vi "report generation  window.vi"(0 "connection reference":T1, 7 "error in":errorcluster) -> (4 "connection reference out":T1, 15 "error out":errorcluster)   [LabVIEW 2024]
uses:
  <vilib>/addons/database/Connection.llb/Conn ObjectReference.ctl
  <vilib>/Utility/miscctls.llb/LVRowAndColumnTypeDef.ctl
  Global variable.vi
  <vilib>/addons/database/Connection.llb/DB Tools Open Connec (String).vi
  Variable/Global.vi
  <vilib>/addons/database/NI_Database_API.lvlib
panel:
  in  "Final Barcode":string
  in  "Search by Laser 2":bool
  in  "Export":bool
  in  "Type of file":enum32{"Text", "Csv"}(radio)
  in  "Report File Name":string
  out "date/time string":string
  out "Result":string[][](table)
  in  "Exit":bool
  in  "Barcode":string
  in  "Search by Date":bool
  in  "model name selection":bool
  in  "MODEL":enum16{"NO Station", "Station 1", "Station 2"}(ring)
  in  "Search by Date":bool
  in  "To Date":timestamp format="%<%y/%m/%d>T"
  in  "From date":timestamp format="%<%y/%m/%d>T"
  out "exit":bool
  out "Numeric":i32
  # "TESTING DATALOGGING SYSTEM"
  # "REPORT SCREEN"
  # "to"
  # "Report  Genrate"
  # "A1234567B567001"
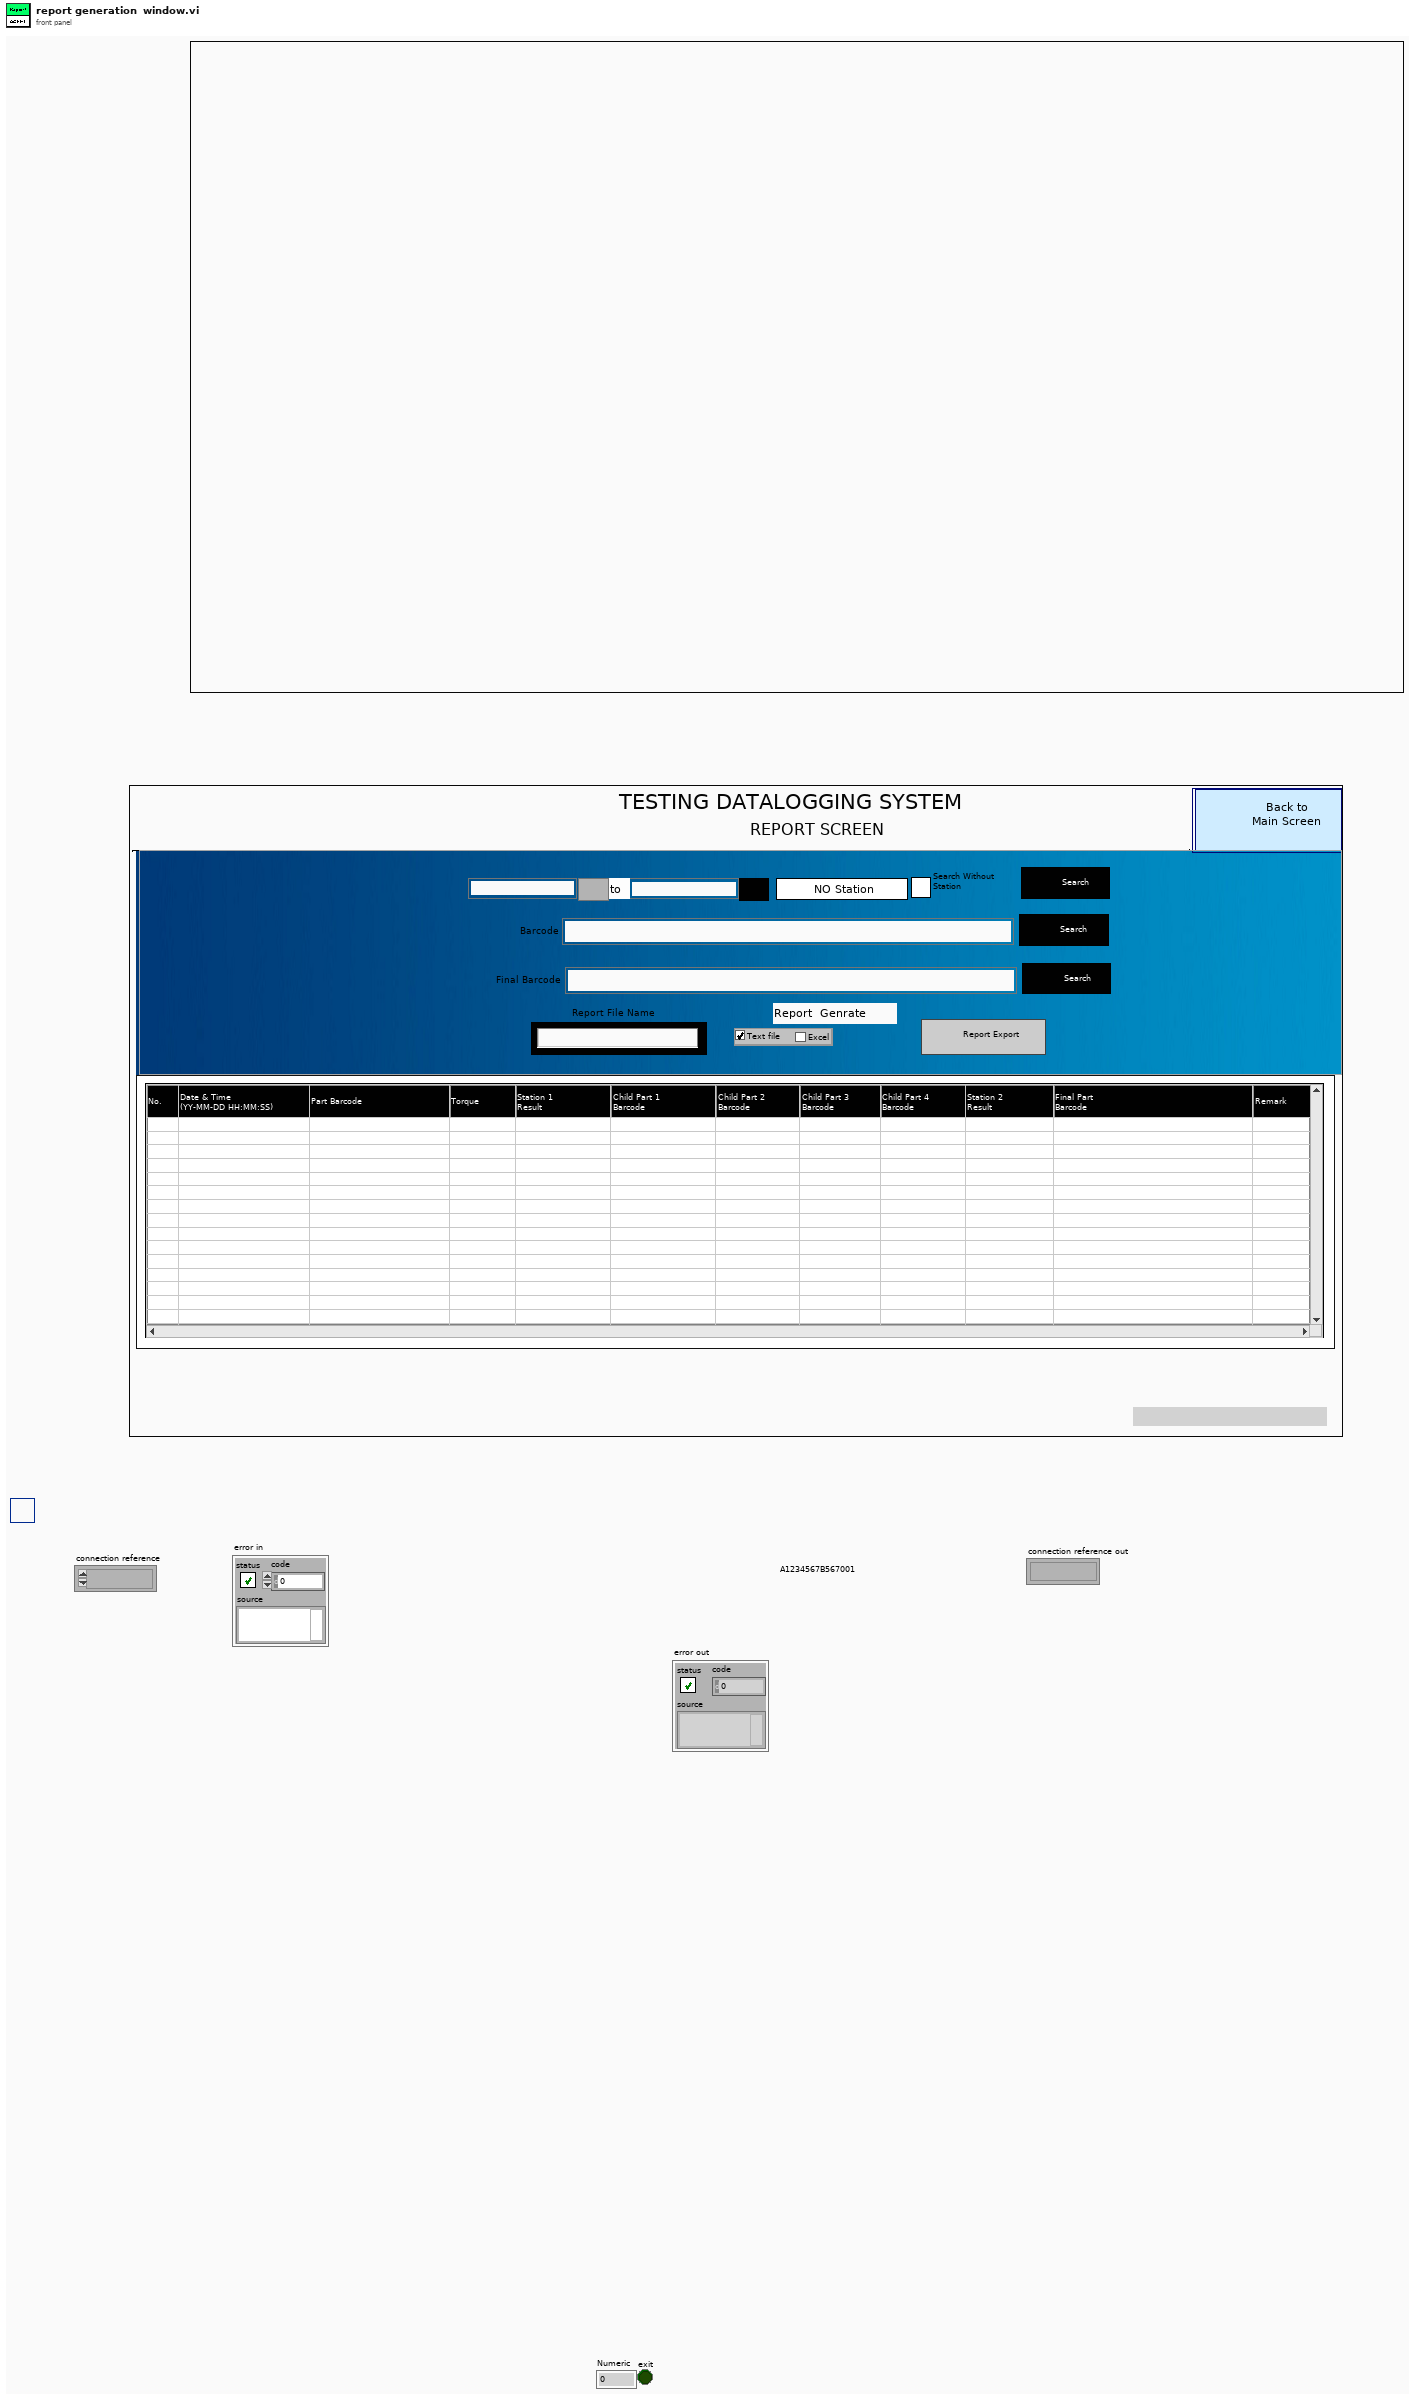
[diagram p1: front panel]
types:
  T1 = typedef "NI_Database_API.lvlib/Conn ObjectReference.ctl" = refnum<k1>
  T2 = typedef "LVRowAndColumnTypeDef.ctl" = cluster{"Row":i32, "Column":i32}
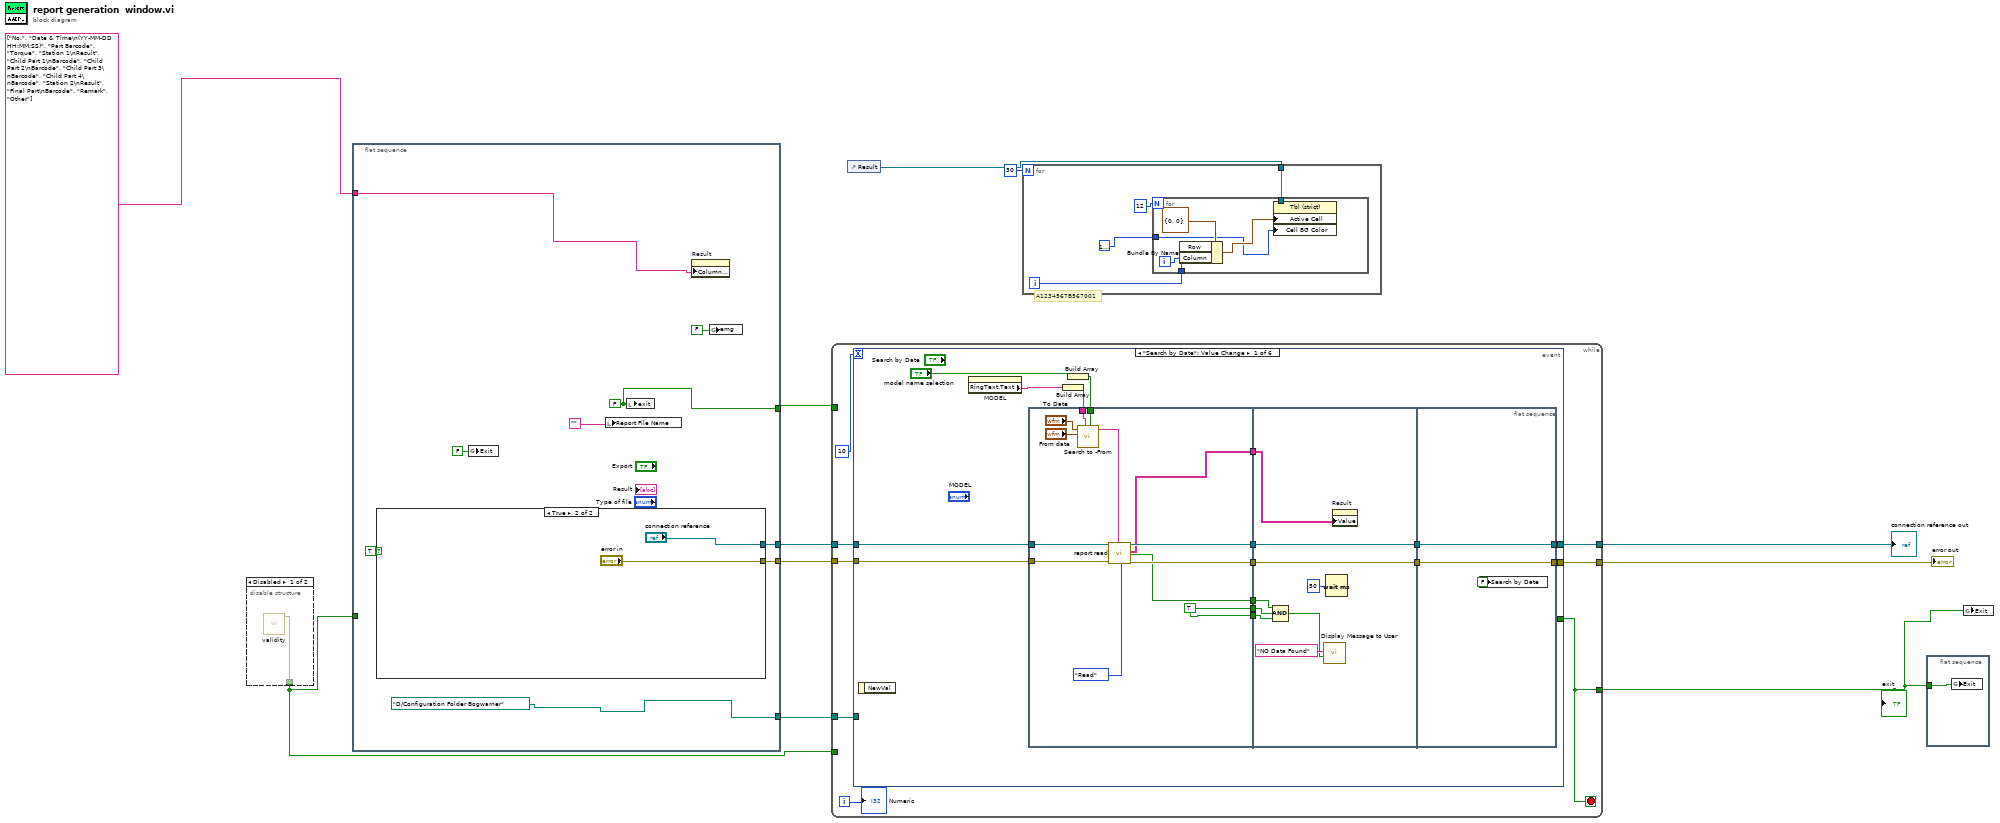
[diagram p0: block diagram]
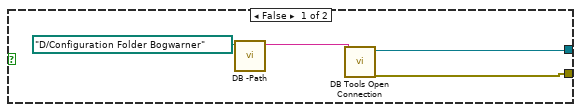
[diagram p3: hidden frame]
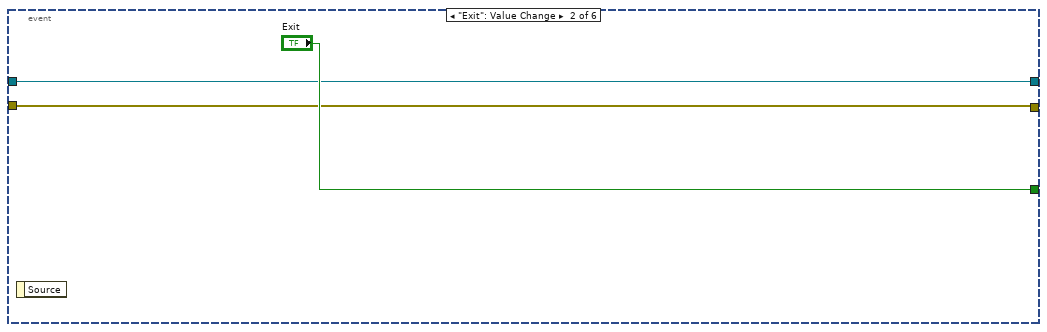
[diagram p4: hidden frame]
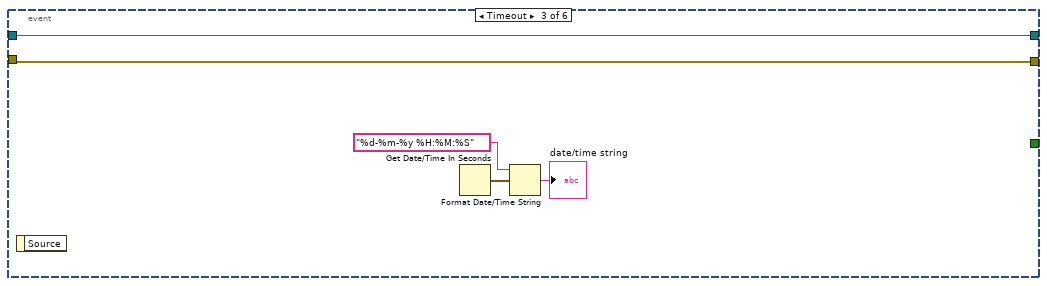
[diagram p5: hidden frame]
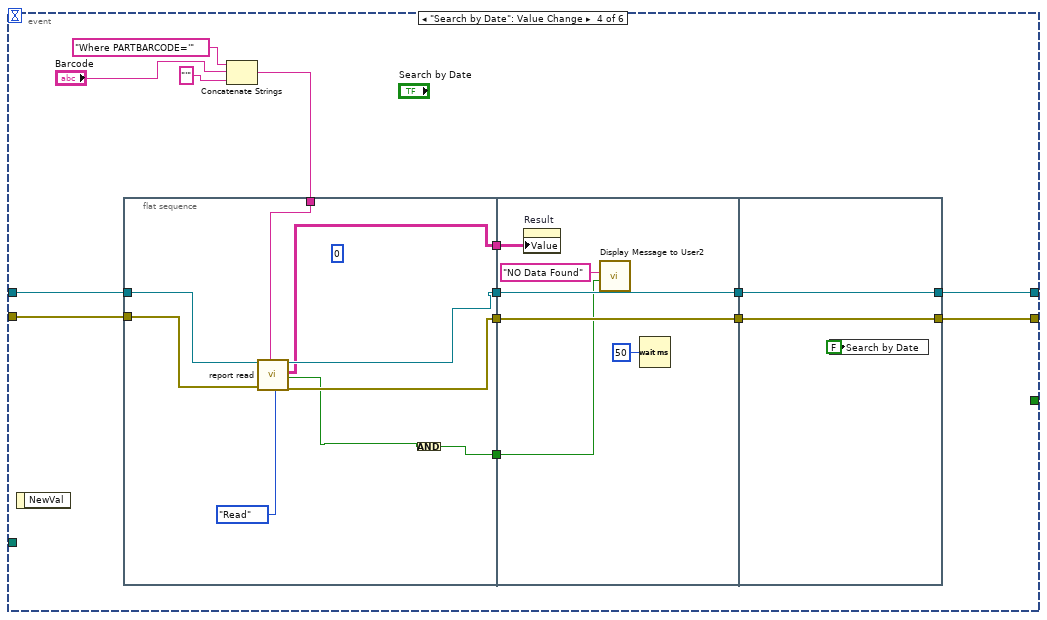
[diagram p6: hidden frame]
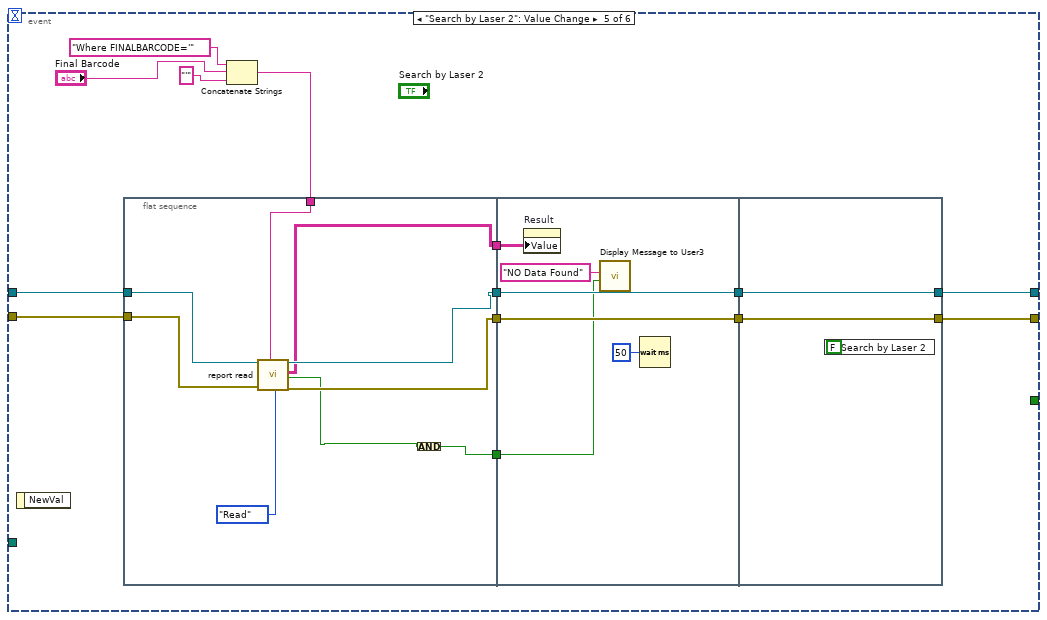
[diagram p7: hidden frame]
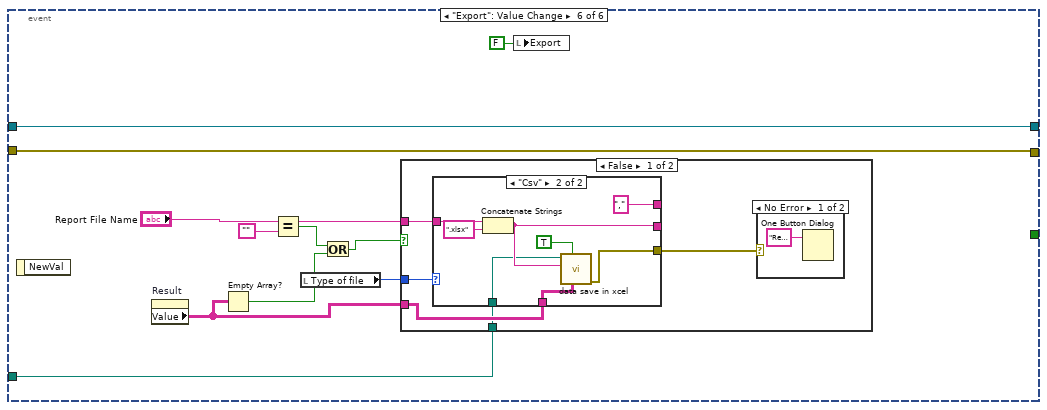
[diagram p8: hidden frame]
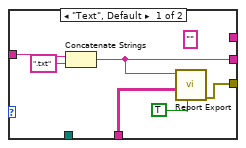
[diagram p10: hidden frame]
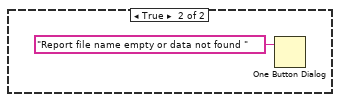
[diagram p11: hidden frame]
diagram:
  # "A1234567B567001"
  n1 = disable-structure shown="Disabled" {
    disable-tunnel: [w12 _] -> w6
    frame Disabled {
      n2 = call "validity.vi"() -> ("NOt valid"=w12:bool)  [unwired: 11 in]
    }
    frame Enabled {
    }
  }
  n3 = flat-sequence {
    tunnel: [w20] -> w10
    tunnel: [w18] -> w8
    tunnel: [w19] -> w7
    tunnel: w6 -> [_]
    tunnel: [path "D:/Configuration Folder Bogwarner" ("path")] -> w4
    tunnel: string[] ["No.", "Date & Time\n(YY-MM-DD HH:MM:SS)", "Part Barcode", "Torque", "Station 1\nResult", "Child Part 1\nBarcode", "Child Part 2\nBarcode", "Child Part 3\nBarcode", "Child Part 4\nBarcode", "Station 2\nResult", "Final Part\nBarcode", "Remark", "Other"] ("Column Header Strings[]") -> [w13]
    frame #0 {
      w20 = FALSE ("exit")
      n4 = case shown="True" TRUE {
        tunnel: [w23 "error in"] -> w19
        tunnel: [w22 "connection reference"] -> w18
        frame False {
          n5 = call "DB -Path.vi"("path"=path "D:/Configuration Folder Bogwarner") -> ("String"=w24:string)  [unwired: 8 in, 2 out]
          n6 = call-poly <vilib>:"DB Tools Open Connection.vi"("connection information"=w24) -> ("error out"=w23:errorcluster, "connection reference"=w22:T1)  [unwired: 7 in]
        }
        frame True {
        }
      }
      n7 = global write "Global variable.vi" "Exit"(FALSE ("Exit")) -> ()
      n8 = local write "Report File Name"("") -> ()
      n9 = local write "exit"(w20) -> ()
      n10 = property on="Result" class="Tbl (strict)"("Column Headers[]"=w13) -> ()  [unwired: 2 in, 2 out]
      n11 = global write "Global.vi" "emg"(FALSE ("emg")) -> ()
    }
  }
  n12 = while {
    tunnel: w8 -> [w35]
    tunnel: w7 -> [w34]
    tunnel: [w33] -> w11
    tunnel: [w32] -> w5
    tunnel: [w31] -> w9
    tunnel: w10 -> [_]
    tunnel: w6 -> [_]
    tunnel: w4 -> [w28]
    i -> [w30]
    stop <- w31 stop-if-true
    n13 = event shown="[0] \"Search by Date\": Value Change" {
      selector: _ -> [_ _ _ _ _ _]
      dyn-events: _ -> [_ _ _ _ _ _]
      timeout: 10 -> [_ _ _ _ _ _]
      tunnel: [_ "Exit" _ _ _ _] -> w31
      tunnel: w35 -> [w51 w78 w84 w98 w130 w159]
      tunnel: w34 -> [w50 w77 w83 w97 w129 w158]
      tunnel: [w49 w78 w84 w96 w128 w159] -> w33
      tunnel: [w48 w77 w83 w95 w127 w158] -> w32
      tunnel: w28 -> [_ _ _ _ _ w149]
      event "Search by Date": Value Change {
        n14 = event-data() -> ()  [unwired: 1 in, 1 out]
        n15 = property on="MODEL" class="Enum (strict)"() -> ("RingText.Text"=w40:string)  [unwired: 2 in, 2 out]
        n16 = flat-sequence {
          tunnel: w51 -> [w64]
          tunnel: w50 -> [w63]
          tunnel: [w60] -> w47
          tunnel: [w59] -> w46
          tunnel: w42 -> [w57]
          tunnel: w41 -> [w56]
          tunnel: [w54] -> w39
          tunnel: [w53] -> w38
          tunnel: [w53] -> w37
          tunnel: [w52] -> w36
          tunnel: w47 -> [w73]
          tunnel: w46 -> [w72]
          tunnel: [w73] -> w45
          tunnel: [w72] -> w44
          tunnel: w39 -> [w68]
          tunnel: w38 -> [w67]
          tunnel: w37 -> [w66]
          tunnel: w36 -> [w69]
          tunnel: [w75] -> w48
          tunnel: [w76] -> w49
          tunnel: w45 -> [w76]
          tunnel: w44 -> [w75]
          frame #0 {
            w53 = TRUE ("DMC TESTED:T")
            n17 = call "Search to -From.vi"("Enable"=w56, "Selection"=w57, "From date"="From date", "To Date"="To Date") -> ("search dataString"=w58:string)  [unwired: 6 in, 1 out]
            n18 = call "report read.vi"("connection reference"=w64, "error in (no error)"=w63, "search dataString"=w58, "Enum"=enum16{"Write", "Read"}."Read") -> ("connection reference out"=w60:T1, "Search result"=w52:string[][], "DMC TESTED:T"=w54:bool, "error out"=w59:errorcluster)  [unwired: 10 in, 2 out]
          }
          frame #1 {
            n19 = Compound Arithmetic op=AND(w68, w67, w66) -> (w65:bool)
            n20 = call "Display Message to User"("Enable"=w65, "Message"="NO Data Found") -> ()  [unwired: 8 in, 2 out]
            n21 = Wait (ms)(milliseconds to wait=u32 50) -> ()  [unwired: 1 out]
            n22 = property on="Result" class="Tbl (strict)"("Value"=w69) -> ()  [unwired: 2 in, 2 out]
          }
          frame #2 {
            n23 = local write "Search by Date"(FALSE ("Search")) -> ()
          }
        }
        n24 = Build Array(w40) -> (w42:string[])
        n25 = Build Array("model name selection") -> (w41:bool[])
      }
      event "Exit": Value Change {
        n26 = event-data() -> ()  [unwired: 1 in, 1 out]
      }
      event Timeout {
        n27 = event-data() -> ()  [unwired: 1 in, 1 out]
        n28 = Get Date/Time In Seconds() -> (seconds since 1Jan1904=w81:timestamp)
        n29 = Format Date/Time String(time format string (%c)="%d-%m-%y %H:%M:%S", seconds (now)=w81) -> (date/time string=→"date/time string":string)  [unwired: 1 in]
      }
      event "Search by Date": Value Change {
        n30 = event-data() -> ()  [unwired: 1 in, 1 out]
        n31 = flat-sequence {
          tunnel: w98 -> [w107]
          tunnel: w97 -> [w106]
          tunnel: [w103] -> w94
          tunnel: [w102] -> w93
          tunnel: w87 -> [w104]
          tunnel: [w100] -> w86
          tunnel: [w99] -> w85
          tunnel: w94 -> [w113]
          tunnel: w93 -> [w112]
          tunnel: [w113] -> w92
          tunnel: [w112] -> w91
          tunnel: w86 -> [w110]
          tunnel: w85 -> [w108]
          tunnel: [w115] -> w95
          tunnel: [w116] -> w96
          tunnel: w92 -> [w116]
          tunnel: w91 -> [w115]
          frame #0 {
            (unwired) 0 ("disabled index (col)")
            n32 = call "report read.vi"("connection reference"=w107, "error in (no error)"=w106, "search dataString"=w104, "Enum"=enum16{"Write", "Read"}."Read") -> ("connection reference out"=w103:T1, "Search result"=w99:string[][], "DMC TESTED:T"=w101:bool, "error out"=w102:errorcluster)  [unwired: 10 in, 2 out]
            n33 = Compound Arithmetic op=AND(w101) -> (w100:bool)
          }
          frame #1 {
            n34 = property on="Result" class="Tbl (strict)"("Value"=w108) -> ()  [unwired: 2 in, 2 out]
            n35 = call "Display Message to User2"("Enable"=w110, "Message"="NO Data Found") -> ()  [unwired: 8 in, 2 out]
            n36 = Wait (ms)(milliseconds to wait=u32 50) -> ()  [unwired: 1 out]
          }
          frame #2 {
            n37 = local write "Search by Date"(FALSE ("Search")) -> ()
          }
        }
        n38 = Concatenate Strings("Where PARTBARCODE='" ("string"), "Barcode", "'" ("string")) -> (w87:string)
      }
      event "Search by Laser 2": Value Change {
        n39 = event-data() -> ()  [unwired: 1 in, 1 out]
        n40 = flat-sequence {
          tunnel: w130 -> [w139]
          tunnel: w129 -> [w138]
          tunnel: [w135] -> w126
          tunnel: [w134] -> w125
          tunnel: w119 -> [w136]
          tunnel: [w132] -> w118
          tunnel: [w131] -> w117
          tunnel: w126 -> [w145]
          tunnel: w125 -> [w144]
          tunnel: [w145] -> w124
          tunnel: [w144] -> w123
          tunnel: w118 -> [w142]
          tunnel: w117 -> [w140]
          tunnel: [w147] -> w127
          tunnel: [w148] -> w128
          tunnel: w124 -> [w148]
          tunnel: w123 -> [w147]
          frame #0 {
            n41 = call "report read.vi"("connection reference"=w139, "error in (no error)"=w138, "search dataString"=w136, "Enum"=enum16{"Write", "Read"}."Read") -> ("connection reference out"=w135:T1, "Search result"=w131:string[][], "DMC TESTED:T"=w133:bool, "error out"=w134:errorcluster)  [unwired: 10 in, 2 out]
            n42 = Compound Arithmetic op=AND(w133) -> (w132:bool)
          }
          frame #1 {
            n43 = property on="Result" class="Tbl (strict)"("Value"=w140) -> ()  [unwired: 2 in, 2 out]
            n44 = call "Display Message to User3"("Enable"=w142, "Message"="NO Data Found") -> ()  [unwired: 8 in, 2 out]
            n45 = Wait (ms)(milliseconds to wait=u32 50) -> ()  [unwired: 1 out]
          }
          frame #2 {
            n46 = local write "Search by Laser 2"(FALSE ("Search")) -> ()
          }
        }
        n47 = Concatenate Strings("Where FINALBARCODE='" ("string"), "Final Barcode", "'" ("string")) -> (w119:string)
      }
      event "Export": Value Change {
        n48 = event-data() -> ()  [unwired: 1 in, 1 out]
        n49 = property on="Result" class="Tbl (strict)"() -> ("Value"=w153:string[][])  [unwired: 2 in, 2 out]
        n50 = Empty Array?(array=w153) -> (empty?=w152:bool)
        n51 = Equal?(x="Report File Name", y="") -> (x = y?=w151:bool)
        n52 = local read "Type of file"() -> (w156:enum32{"Text", "Csv"})
        n53 = Or(x=w151, y=w152) -> (x .or. y?=w150:bool)
        n54 = case shown="False" w150 {
          tunnel: w156 -> [w164 _]
          tunnel: "Report File Name" -> [w163 _]
          tunnel: w153 -> [w162 _]
          tunnel: w149 -> [w160 _]
          frame False {
            n55 = case shown="\"Csv\"" w164 {
              tunnel: w163 -> [w171 w178]
              tunnel: [w168 w175] -> _
              tunnel: [_ "," ("string")] -> _
              tunnel: w162 -> [w167 w174]
              tunnel: [w166 w173] -> w161
              tunnel: w160 -> [_ w172]
              frame "Text", Default {
                (unwired) ""
                n56 = Concatenate Strings(w171, ".txt" ("string")) -> (w168:string)
                n57 = call "Report Export.vi"("Condition"=TRUE, "Data"=w167, "Report Type"=w168) -> ("error out"=w166:errorcluster)  [unwired: 7 in]
              }
              frame "Csv" {
                n58 = Concatenate Strings(w178, ".xlsx" ("string")) -> (w175:string)
                n59 = call "data save in xcel.vi"("Data"=w174, "Condition"=TRUE, "Report Type"=w175, "Temp Path"=w172) -> ("error out"=w173:errorcluster)  [unwired: 7 in]
              }
            }
            n60 = case shown="No Error" w161 {
              frame No Error {
                n61 = One Button Dialog(message="Report saved ") -> ()  [unwired: 1 in, 1 out]
              }
              frame Error {
              }
            }
          }
          frame True {
            n62 = One Button Dialog(message="Report file name empty or data not found ") -> ()  [unwired: 1 in, 1 out]
          }
        }
        n63 = local write "Export"(FALSE ("Export")) -> ()
      }
    }
    "Numeric" <- w30
  }
  "error out" <- w5
  "exit" <- w9
  "connection reference out" <- w11
  n64 = control-ref of="Result"() -> (w3:refnum<vi>)
  n65 = for {
    N: 30 -> [_]
    tunnel: w3 -> [w182]
    i -> [w184]
    n66 = for {
      N: 12 -> [_]
      tunnel: w184 -> [w189]
      tunnel: u32 16777225 -> [w185]
      tunnel: w182 -> [w187]
      i -> [w188]
      n67 = Bundle By Name(cluster=T2 {"Row"=0, "Column"=0} ("Active Cell:Active Cell"), "Row"=w189, "Column"=w188) -> (w186:T2)
      n68 = property class="Tbl (strict)"(reference=w187, "Active Cell"=w186, "Cell BG Color"=w185) -> ()  [unwired: 1 in, 2 out]
    }
  }
  n69 = flat-sequence {
    tunnel: w9 -> [w191]
    frame #0 {
      n70 = global write "Global.vi" "Exit"(w191) -> ()
    }
  }
  n71 = global write "Global variable.vi" "Exit"(w9) -> ()
